vi "Temp Calibration.vi"() -> ()   [LabVIEW 2015]
panel:
  in  "Numeric":i32
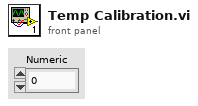
[diagram p1: front panel]
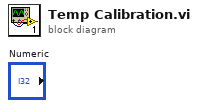
[diagram p0: block diagram]
diagram:
